vi "check if over time cutoff.vi"(11 "cutoff time":timestamp) -> (3 "past due?":bool)   [LabVIEW 2018]
panel:
  out "current time":timestamp
  out "current time double":dbl format="%#_16g"
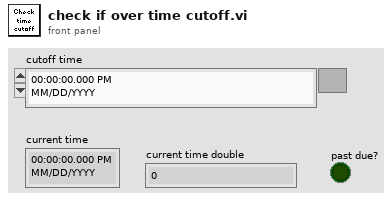
[diagram p1: front panel]
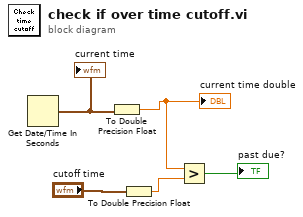
[diagram p0: block diagram]
diagram:
  n1 = Get Date/Time In Seconds() -> (seconds since 1Jan1904=w5:timestamp)
  "current time" <- w5
  n2 = To Double Precision Float(number=w5) -> (double precision float=w3:dbl)
  "current time double" <- w3
  n3 = To Double Precision Float(number="cutoff time") -> (double precision float=w2:dbl)
  n4 = Greater?(x=w3, y=w2) -> (0:→"past due?":bool)
